vi "Create and Start.vi"(6 "Worker Alias":string="Message Pump", 7 "Caller":refnum<class "Worker.lvclass">, 8 "error in (no error)":errorcluster, 9 "Period (ms)":i32=-1, 10 "Time Elapsed Response Case (Case Label)":T1, 11 "Message Pump in":refnum<class "Message Pump.lvclass">) -> (0 "error out":errorcluster, 3 "Message Pump out":refnum<class "Message Pump.lvclass">, 5 "dup Caller out":refnum<class "Worker.lvclass">)   [LabVIEW 2017, in "Message Pump.lvclass"]
doc: "<b>Note: For ease of use, this VI is a wrapper around this Worker's standard Public API VIs. You can also use this Worker's Public API VIs in its place.</b>\n\nDynamically launches and starts an instance of the Message Pump Worker. The Message Pump Worker uses the timeout of an Event Structure to send messages at a fixed interval in the form of a Public API Response.\n\n-----------\n\n<b>Inputs ></b>\n\n<b>Time Elapsed Response Case (Case Label)</b>: The case of <b>Caller</b> that will receive the pumped message.\n\n<b>Period (ms)</b>: The wait time in milliseconds between pumped messages. 20 ms is the minimum possible wait time. A value of -1 will stop messages from being pumped.\n\n<b>Worker Alias</b>: The name of the message pump. This name is local to the Worker it is called from. This input is required if multiple Message Pumps are to be used by the calling Worker."
uses:
  Message Pump.lvclass
  <vilib>/addons/_Workers/Library/Classes/Worker/Worker.lvclass
  <vilib>/addons/_Workers/Library/Case Label.ctl
  Initialization Data.ctl
  Response Cases.ctl
  rqp_Set EHL Timeout.ctl
  <vilib>/addons/_Workers/Library/Workers.lvlib
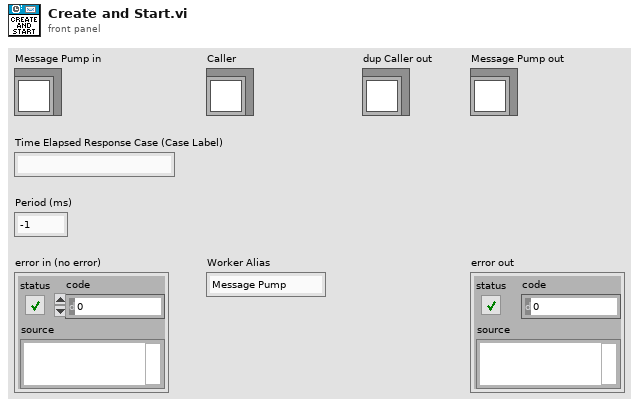
[diagram p1: front panel]
types:
  T1 = typedef "WORKERS.lvlib/Case Label.ctl" = string
  T2 = typedef "Message Pump.lvclass/rqp_Set EHL Timeout.ctl" = cluster{"Timeout (ms)":i32}
  T3 = typedef "Message Pump.lvclass/Initialization Data.ctl" = cluster{"Response Cases":T4}
  T4 = typedef "Message Pump.lvclass/Response Cases.ctl" = cluster{"Timer Elapsed":T5}
  T5 = typedef "Workers.lvlib/Case Label.ctl" = string
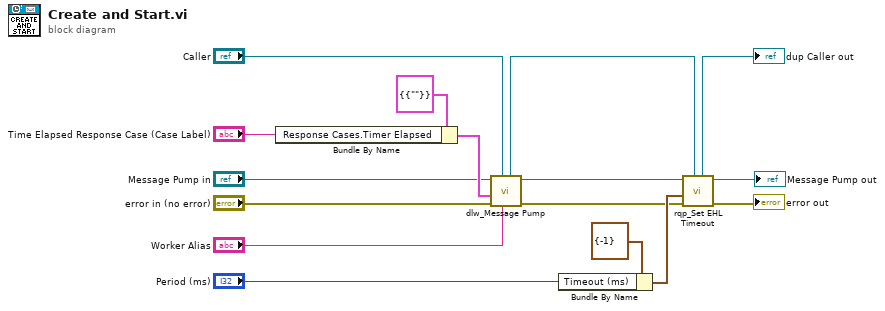
[diagram p0: block diagram]
diagram:
  n1 = Bundle By Name(cluster=T3 {"Response Cases"={"Timer Elapsed"=""}} ("Initialization Data"), "Response Cases.Timer Elapsed"="Time Elapsed Response Case (Case Label)") -> (w14:T3)
  n2 = call "dlw_Message Pump.vi"("Worker Alias"="Worker Alias", "Caller in"="Caller", "error in"="error in (no error)", "Initialization Data"=w14, "Message Pump in"="Message Pump in") -> ("error out"=w4:errorcluster, "Message Pump out"=w8:refnum<class "Message Pump.lvclass">, "dup Caller out"=w10:refnum<class "Worker.lvclass">)  [unwired: 4 in]
  n3 = Bundle By Name(cluster=T2 {"Timeout (ms)"=-1} ("Data in"), "Timeout (ms)"="Period (ms)") -> (w6:T2)
  n4 = call "rqp_Set EHL Timeout.vi"("Caller in"=w10, "error in"=w4, "Data in"=w6, "Message Pump in"=w8) -> ("error out"=→"error out":errorcluster, "dup Message Pump out"=→"Message Pump out":refnum<class "Message Pump.lvclass">, "dup Caller out"=→"dup Caller out":refnum<class "Worker.lvclass">)  [unwired: 5 in]
